vi "SetValueByItemIndex.vi"(0 "VI Reference In":refnum<vi>, 2 "delimiter (>>)":string=">>", 5 "Control Path":string, 7 "Item Index":i32, 11 "Error In":errorcluster) -> (4 "VI Reference Out":refnum<vi>, 15 "Error Out":errorcluster)   [LabVIEW 2016, in "Drona.lvlib" / "ControlValue.lvlib" / "StimulusMCListbox.lvlib"]
doc: "Sets value(signaling) for the multi column listbox control whose index is specified. \n\nThe input control name is given as a string , incase of path, use delimiters inbetween the path."
uses:
  StimulusMCListbox.lvlib
  <vilib>/Utility/error.llb/Error Cluster From Error Code.vi
  <vilib>/ErrorRing/Error Ring.xnode
  Drona.lvlib
  Get/GetControlRef/GetControlRef.lvlib
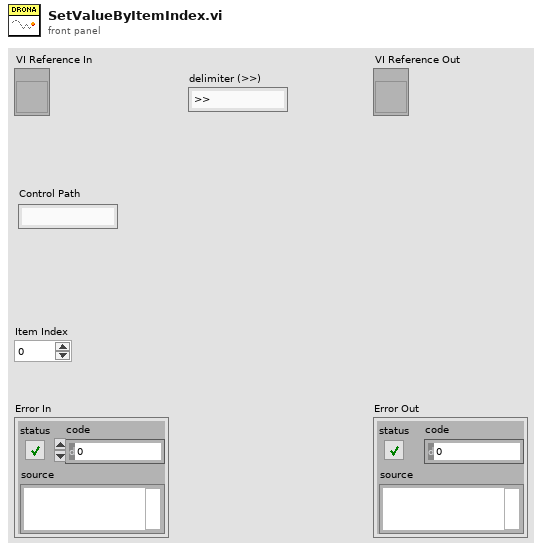
[diagram p1: front panel]
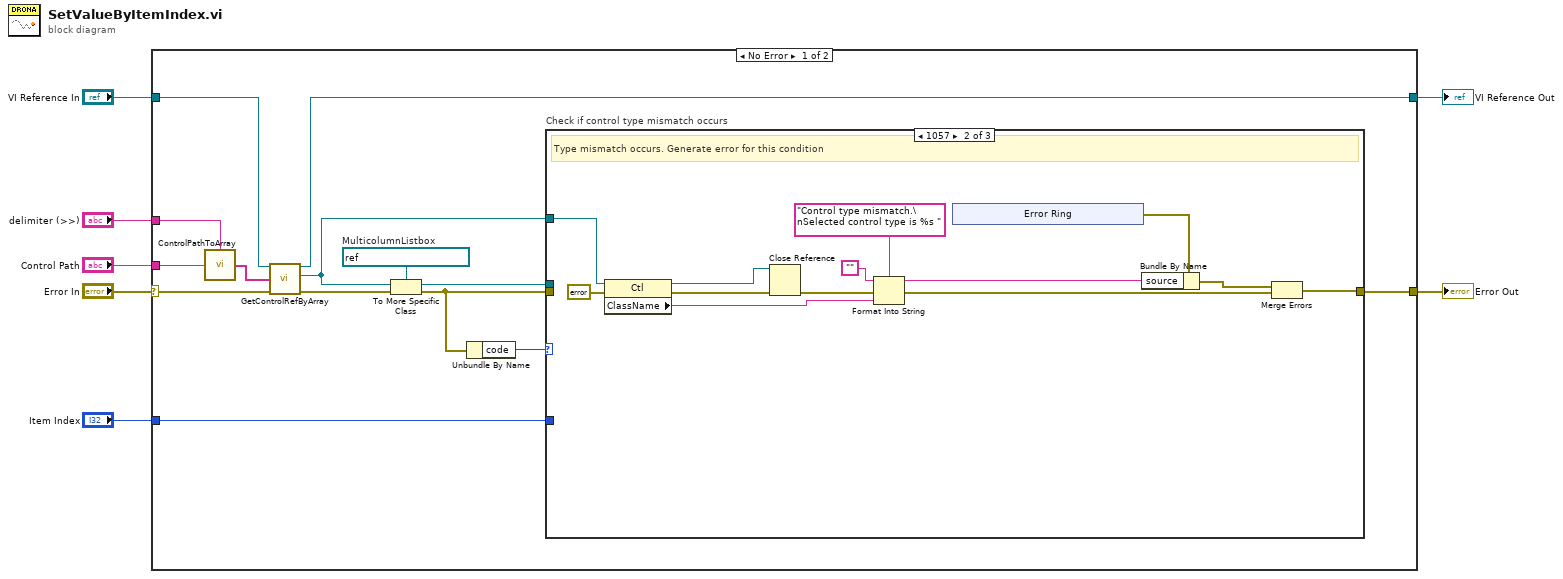
[diagram p0: block diagram]
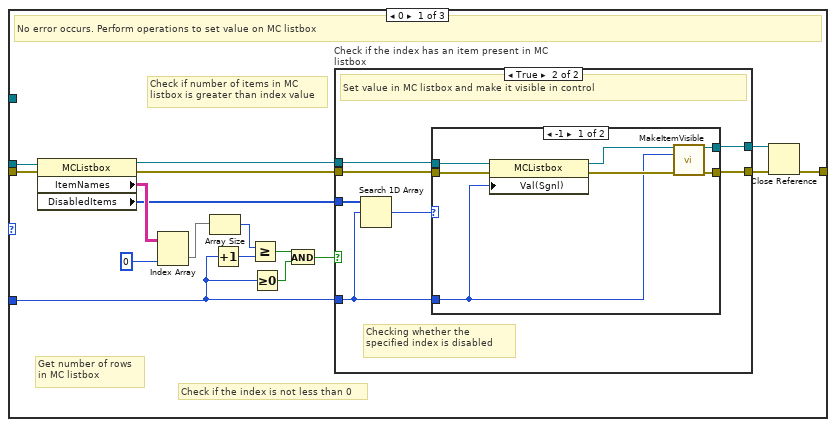
[diagram p2: hidden frame]
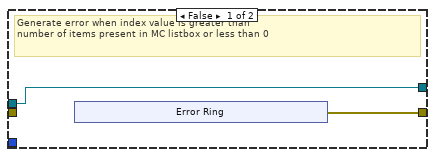
[diagram p3: hidden frame]
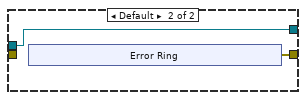
[diagram p4: hidden frame]
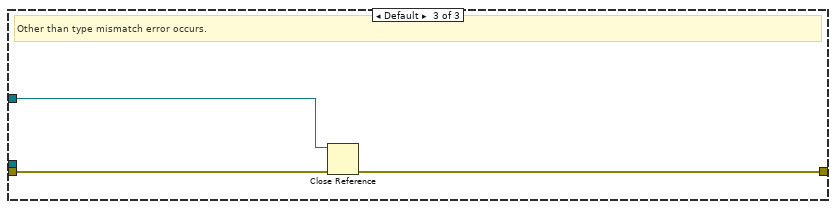
[diagram p5: hidden frame]
diagram:
  n1 = case shown="No Error" "Error In" {
    selector: "Error In" -> [w10 w89]
    tunnel: [w18 w89] -> w6
    tunnel: "VI Reference In" -> [w14 w88]
    tunnel: "Control Path" -> [w20 _]
    tunnel: "Item Index" -> [w16 _]
    tunnel: [w13 w88] -> w2
    tunnel: "delimiter (>>)" -> [w19 _]
    frame No Error {
      w21 = refnum<vi> refnum  # MulticolumnListbox
      n2 = call "ControlPathToArray.vi"("Control Name"=w20, "delimiter (>>)"=w19) -> ("Control Path"=w15:string[])
      n3 = call "GetControlRefByArray.vi"("VI Reference In"=w14, "Control Path"=w15, "error In"=w10) -> ("VI Reference Out"=w13:refnum<vi>, "Ctl Refnum"=w11:refnum<vi>, "error out"=w12:errorcluster)  [unwired: 10 in]
      n4 = To More Specific Class(target class=w21, reference=w11, error in=w12) -> (specific class reference=w17:refnum<vi>, error out=w9:errorcluster)
      n5 = Unbundle By Name(w9) -> ("code"=w8:i32)
      n6 = case "Check if control type mismatch occurs" shown="1057" w8 {
        tunnel: [w38 w69 w86] -> w18
        tunnel: w17 -> [w31 _ _]
        tunnel: w16 -> [w29 _ _]
        tunnel: w11 -> [_ w79 w85]
        tunnel: w9 -> [w37 _ w87]
        frame 0 {
          # "Get number of rows\nin MC listbox"
          # "Check if the index is not less than 0"
          # "Check if number of items in MC \nlistbox is greater than index value"
          # "No error occurs. Perform operations to set value on MC listbox"
          n7 = property class="MCListbox"(reference=w31, error in=w37) -> (reference out=w30:refnum<vi>, error out=w34:errorcluster, "ItemNames"=w28:string[][], "DisabledItems"=w22:i32[])
          n8 = Index Array(array=w28, index (col)=0 ("disabled index (col)")) -> (element=w27:string[])  [unwired: 1 in]
          n9 = Array Size(array=w27) -> (size(s)=w33:i32)
          n10 = Increment(x=w29) -> (x+1=w32:i32)
          n11 = Greater Or Equal?(x=w33, y=w32) -> (x >= y?=w26:bool)
          n12 = Greater Or Equal To 0?(x=w29) -> (x >= 0?=w25:bool)
          n13 = And(x=w26, y=w25) -> (x .and. y?=w24:bool)
          n14 = case "Check if the index has an item present in MC listbox" shown="True" w24 {
            tunnel: [w39 w49] -> w36
            tunnel: [w40 w50] -> w35
            tunnel: w34 -> [_ w52]
            tunnel: w30 -> [w40 w51]
            tunnel: w29 -> [_ w47]
            tunnel: w22 -> [_ w48]
            frame False {
              # "Generate error when index value is greater than \nnumber of items present in MC listbox or less than 0"
              n15 = xnode "Error Ring"() -> ("error out"=w39:errorcluster)
            }
            frame True {
              # "Checking whether the specified index is disabled"
              # "Set value in MC listbox and make it visible in control"
              n16 = Search 1D Array(1D array=w48, element=w47) -> (index of element=w46:i32)  [unwired: 1 in]
              n17 = case shown="-1" w46 {
                tunnel: w52 -> [w59 _]
                tunnel: w51 -> [w58 w61]
                tunnel: w47 -> [w55 _]
                tunnel: [w54 w61] -> w50
                tunnel: [w53 w60] -> w49
                frame -1 {
                  n18 = property class="MCListbox"(reference=w58, error in=w59, "Val(Sgnl)"=w55) -> (reference out=w56:refnum<vi>, error out=w57:errorcluster)
                  n19 = call "MakeItemVisible.vi"("MC ListBox Ref In"=w56, "Item Index"=w55, "Error In"=w57) -> ("MC ListBox Ref Out"=w54:refnum<vi>, "Error Out"=w53:errorcluster)  [unwired: 11 in]
                }
                frame Default {
                  n20 = xnode "Error Ring"() -> ("error out"=w60:errorcluster)
                }
              }
            }
          }
          n21 = Close Reference(reference=w35, error in (no error)=w36) -> (error out=w38:errorcluster)
        }
        frame 1057 {
          # "Type mismatch occurs. Generate error for this condition"
          n22 = property class="Ctl"(reference=w79, error in=errorcluster {"status"=FALSE, "code"=0, "source"=""} ("error out")) -> (reference out=w67:refnum<vi>, error out=w78:errorcluster, "ClassName"=w75:string)
          n23 = Close Reference(reference=w67, error in (no error)=w78) -> (error out=w68:errorcluster)
          n24 = Format Into String(format string="Control type mismatch.\nSelected control type is %s ", initial string="", error in=w68, w75) -> (resulting string=w72:string, error out=w70:errorcluster)
          n25 = xnode "Error Ring"() -> ("error out"=w73:errorcluster)
          n26 = Bundle By Name(cluster=w73, "source"=w72) -> (w71:errorcluster)
          n27 = Merge Errors(w71, w70) -> (w69:errorcluster)
        }
        frame Default {
          # "Other than type mismatch error occurs."
          n28 = Close Reference(reference=w85, error in (no error)=w87) -> (error out=w86:errorcluster)
        }
      }
    }
    frame Error {
    }
  }
  "Error Out" <- w6
  "VI Reference Out" <- w2
